vi "read.vi"(8 "error in (no error)":errorcluster, 9 "timeout (s)":i32=1000, 10 "buffer size":i32=1000, 11 "Telnet in":refnum<class "Telnet.lvclass">) -> (0 "error out":errorcluster, 1 "finished":bool, 2 "read":string, 3 "Telnet out":refnum<class "Telnet.lvclass">)   [LabVIEW 2011, in "Hardware.lvlib" / "HWControllers.lvlib" / "Telnet.lvclass"]
uses:
  Telnet.lvclass
  Telnet.lvclass/Telnet.ctl
  <vilib>/addons/internet/NI_InternetTK_Core_VIs.lvlib
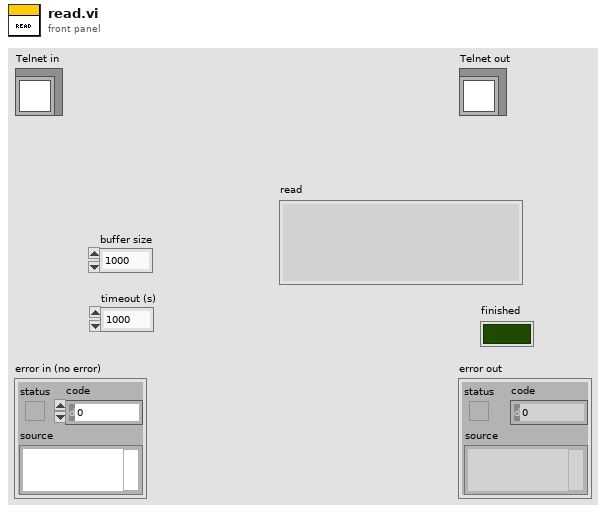
[diagram p1: front panel]
types:
  T1 = typedef "Telnet Session.ctl" = refnum<k1>
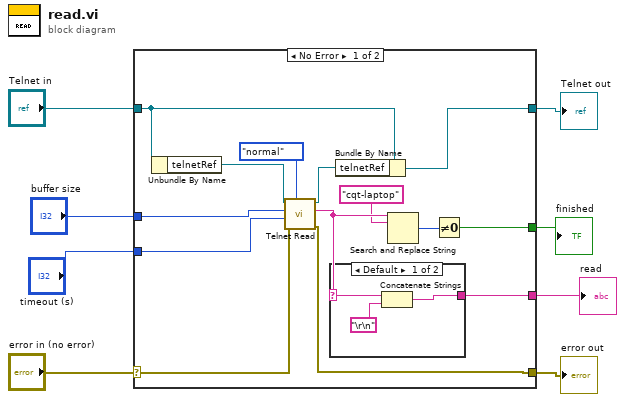
[diagram p0: block diagram]
diagram:
  n1 = case shown="No Error" "error in (no error)" {
    selector: "error in (no error)" -> [w14 w27]
    tunnel: [w13 w27] -> w7
    tunnel: [w16 w26] -> w5
    tunnel: "Telnet in" -> [w17 w26]
    tunnel: "buffer size" -> [w20 _]
    tunnel: [w19 _] -> w3
    tunnel: "timeout (s)" -> [w15 _]
    tunnel: [w9 _] -> w1
    frame No Error {
      n2 = Unbundle By Name(w17) -> ("telnetRef"=w21:T1)
      n3 = call <vilib>:"Telnet Read.vi"("read mode (normal)"=enum16{"normal", "line", "buffered"}."normal", "error in (no error)"=w14, "timeout ms (25000)"=w15, "bytes to read"=w20, "telnet connection"=w21) -> ("error out"=w13:errorcluster, "data out"=w12:string, "telnet connection out"=w18:T1)  [unwired: 2 out]
      n4 = case shown="Default" w12 {
        selector: w12 -> [w25 _]
        tunnel: [w23 _] -> w19
        frame Default {
          n5 = Concatenate Strings(w25, "\r\n") -> (w23:string)
        }
        frame "" {
        }
      }
      n6 = Bundle By Name(cluster=w17, "telnetRef"=w18) -> (w16:refnum<class "Telnet.lvclass">)
      n7 = Search and Replace String(input string=w12, search string="cqt-laptop") -> (number of replacements=w10:i32)  [unwired: 6 in, 3 out]
      n8 = Not Equal To 0?(x=w10) -> (x != 0?=w9:bool)
    }
    frame Error {
    }
  }
  "error out" <- w7
  "Telnet out" <- w5
  "read" <- w3
  "finished" <- w1
